vi "odomPos.vi"(2 "encoderCounts":cluster{"dRight":i32, "dLeft":i32}, 3 "posInput":cluster{"xPos":dbl, "yPos":dbl, "Theta":dbl}) -> (1 "posOutput":cluster{"xPos":dbl, "yPos":dbl, "Theta":dbl})   [LabVIEW 2016]
uses:
  <vilib>/Analysis/coordinate.llb/Angle Units.ctl
  <vilib>/Analysis/coordinate.llb/Angle Range (Degree).ctl
  <vilib>/Analysis/coordinate.llb/Wrap Angle (scalar).vi
  <vilib>/Analysis/NI_AAL_Angle.lvlib
panel:
  in  "wheelDia":dbl=100.0
  in  "width":dbl=271.0
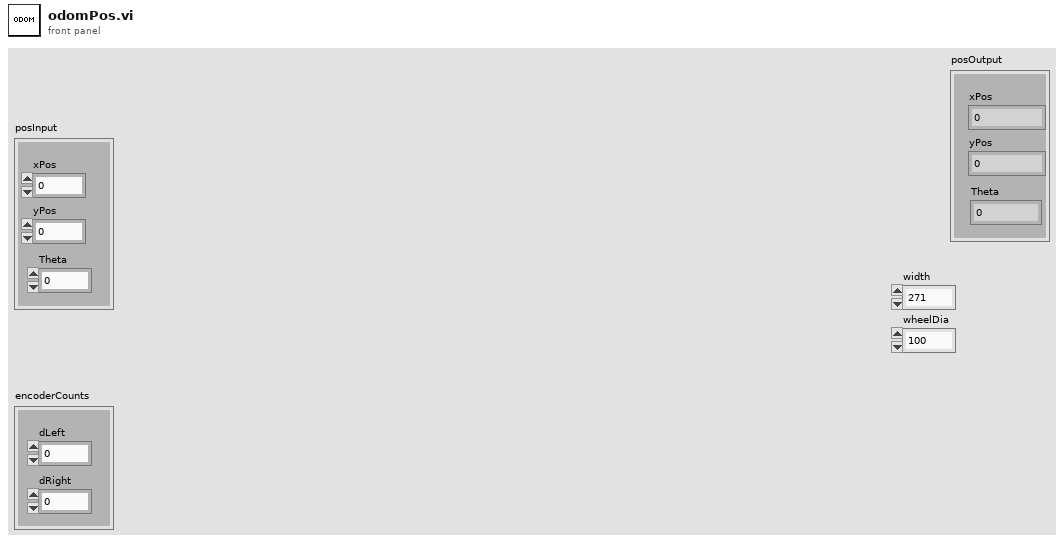
[diagram p1: front panel]
types:
  T1 = typedef "NI_AAL_Angle.lvlib/Angle Range (Degree).ctl" = u16
  T2 = typedef "NI_AAL_Angle.lvlib/Angle Units.ctl" = i32
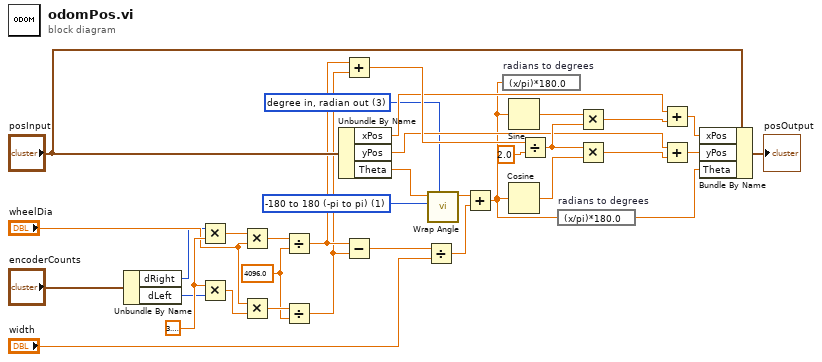
[diagram p0: block diagram]
diagram:
  w7 = T1 1 items=["none", "-180 to 180 (-pi to pi)", "0 to 360 (0 to 2pi)"] ("angle range")
  w5 = T2 3 items=["radian in, radian out", "radian in, degree out", "degree in, degree out", "degree in, radian out"] ("angle units")
  w9 = 4096.0 ("y")
  w32 = 3.141592653589793
  n1 = Unbundle By Name("encoderCounts") -> ("dRight"=w15:i32, "dLeft"=w16:i32)
  n2 = Multiply(x=w15, y=w32) -> (x*y=w33:dbl)
  n3 = Multiply(x=w32, y=w16) -> (x*y=w34:dbl)
  n4 = Multiply(x=w33, y="wheelDia") -> (x*y=w10:dbl)
  n5 = Multiply(x="wheelDia", y=w34) -> (x*y=w11:dbl)
  n6 = Divide(x=w10, y=w9) -> (x/y=w2:dbl)
  n7 = Divide(x=w11, y=w9) -> (x/y=w1:dbl)
  n8 = Unbundle By Name("posInput") -> ("xPos"=w22:dbl, "yPos"=w20:dbl, "Theta"=w4:dbl)
  n9 = Add(x=w2, y=w1) -> (x+y=w28:dbl)
  n10 = Subtract(x=w2, y=w1) -> (x-y=w8:dbl)
  n11 = Divide(x=w8, y="width") -> (x/y=w29:dbl)
  n12 = call-poly <vilib>:"Wrap Angle.vi"("angle units"=w5, "angle range"=w7, "angle in"=w4) -> ("angle out"=w3:dbl)  [unwired: 7 in, 1 out]
  n13 = Add(x=w3, y=w29) -> (x+y=w6:dbl)
  n14 = expression code="(x/pi)*180.0" "radians to degrees"(w6) -> ()  [unwired: 1 out]
  n15 = Sine(x=w6) -> (sin(x)=w26:dbl)
  n16 = Cosine(x=w6) -> (cos(x)=w25:dbl)
  n17 = Divide(x=w28, y=2.0) -> (x/y=w24:dbl)
  n18 = expression code="(x/pi)*180.0" "radians to degrees"(w6) -> (w12:dbl)
  n19 = Multiply(x=w26, y=w24) -> (x*y=w23:dbl)
  n20 = Multiply(x=w24, y=w25) -> (x*y=w21:dbl)
  n21 = Add(x=w22, y=w23) -> (x+y=w18:dbl)
  n22 = Add(x=w20, y=w21) -> (x+y=w19:dbl)
  n23 = Bundle By Name(cluster="posInput", "xPos"=w18, "yPos"=w19, "Theta"=w12) -> (→"posOutput":cluster{"xPos":dbl, "yPos":dbl, "Theta":dbl})
